vi "Create New Record in Recordset.vi"(4 "Field Names":variant[](array[variant]), 5 "Field Values":variant[](array[variant]), 6 "error in (no error)":errorcluster, 9 "Recordset":refnum<k7>) -> (0 "error out":errorcluster, 3 "Recordset Out":refnum<k7>)   [LabVIEW 2014, in "hse-db.lvlib" / "ADO-DB-Driver.lvlib"]
uses:
  ADO-DB-Driver.lvlib
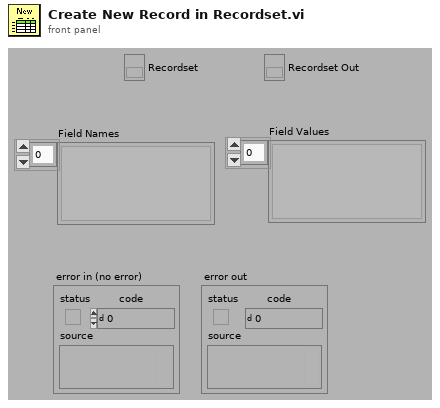
[diagram p1: front panel]
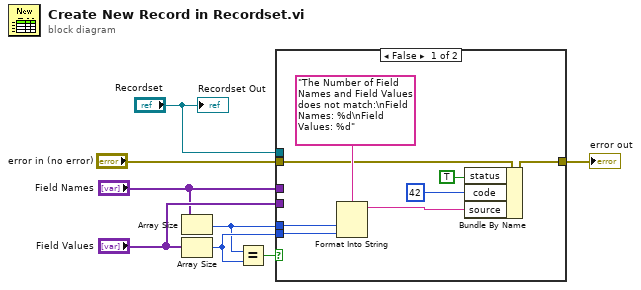
[diagram p0: block diagram]
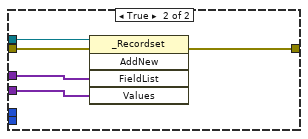
[diagram p2: hidden frame]
diagram:
  n1 = Array Size(array="Field Names") -> (size(s)=w2:i32)
  n2 = Array Size(array="Field Values") -> (size(s)=w3:i32)
  n3 = Equal?(x=w2, y=w3) -> (x = y?=w6:bool)
  n4 = case shown="False" w6 {
    tunnel: "error in (no error)" -> [w13 w21]
    tunnel: [w11 w20] -> w1
    tunnel: "Field Values" -> [_ w19]
    tunnel: "Field Names" -> [_ w18]
    tunnel: "Recordset" -> [_ w17]
    tunnel: w3 -> [w15 _]
    tunnel: w2 -> [w16 _]
    frame False {
      n5 = Format Into String(format string="The Number of Field Names and Field Values does not match:\nField Names: %d\nField Values: %d", w16, w15) -> (resulting string=w12:string)  [unwired: 2 in, 1 out]
      n6 = Bundle By Name(cluster=w13, "status"=TRUE ("Halt?"), "code"=42, "source"=w12) -> (w11:errorcluster)
    }
    frame True {
      n7 = invoke class="_Recordset" method="AddNew"(reference=w17, error in=w21, "FieldList"=w18, "Values"=w19) -> (error out=w20:errorcluster)  [unwired: 1 in, 4 out]
    }
  }
  "error out" <- w1
  "Recordset Out" <- "Recordset"
